vi "Set IPS Action.vi"(8 "error in (no error)":errorcluster, 10 "PSU Act Stat":T1="HOLD" caption="PSU Action Status", 11 "Instrument.Oxford1820 in":refnum<class "Instrument.Oxford1820.lvclass">) -> (0 "error out":errorcluster, 2 "Response":string, 3 "Instrument.Oxford1820 out":refnum<class "Instrument.Oxford1820.lvclass">)   [LabVIEW 2019, in "Instrument.Oxford1820.lvclass"]
uses:
  Instrument.Oxford1820.lvclass
  <instrlib>/Mercury iXX/Public/Libraries/Magnet/Controls/PSU Actions.ctl
  Instrument.Oxford1820.lvclass/Instrument.Oxford1820.ctl
  <instrlib>/Mercury iXX/Public/Libraries/Magnet/Open/Open Magnet Device.vi
  <instrlib>/Mercury iXX/Public/Libraries/Magnet/Configuration/Set/PSU Action Status (Set).vi
  <instrlib>/Mercury iXX/Public/Libraries/Magnet/Configuration/Read/PSU Action Status (Read).vi
  <instrlib>/Mercury iXX/Mercury iXX.lvlib
  <instrlib>/Mercury iXX/Public/Libraries/Magnet.lvlib
panel:
  out "Numeric":i32
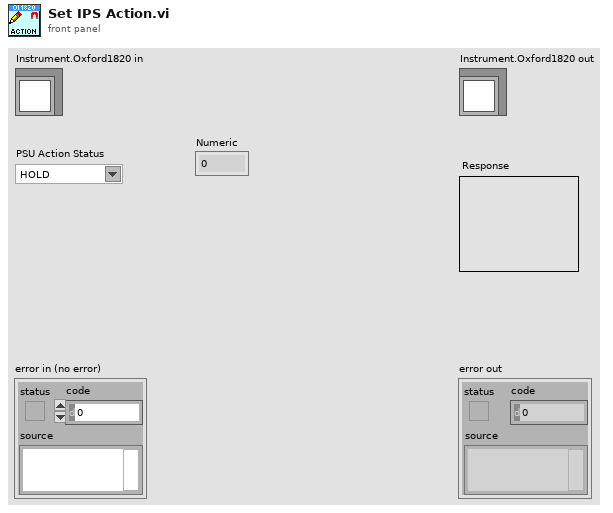
[diagram p1: front panel]
types:
  T1 = typedef "Mercury iXX.lvlib/Magnet.lvlib/PSU Actions.ctl" = string
  T2 = typedef "Mercury iXX.lvlib/Mercury Reference.ctl" = cluster{"Comms":refnum<visa-resource-name>, "Device ID":string[], "Comms Layer":T3, "Command":string, "Query reference":T4}
  T3 = typedef "Mercury iXX.lvlib/Comms Transport Layer.ctl" = enum16{"Ethernet TCP/IP", "USB", "ISOBus - RS-232", "GPIB"}
  T4 = typedef "Mercury iXX.lvlib/Query Dynamic Reference.ctl" = refnum<vi>
  T5 = typedef "Mercury iXX.lvlib/Response String.ctl" = string
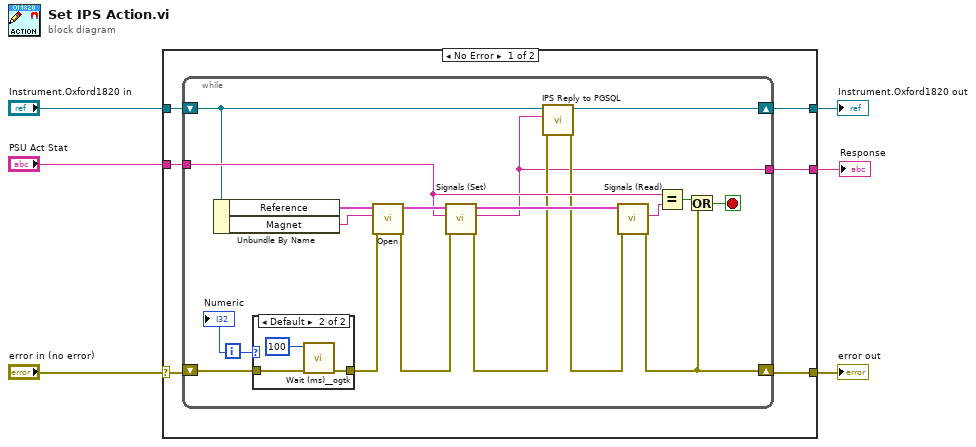
[diagram p0: block diagram]
diagram:
  n1 = case shown="No Error" "error in (no error)" {
    selector: "error in (no error)" -> [w11 w36]
    tunnel: [w9 w36] -> w5
    tunnel: [w7 w35] -> w3
    tunnel: "Instrument.Oxford1820 in" -> [w12 w35]
    tunnel: [w10 _] -> w2
    tunnel: "PSU Act Stat" -> [w8 _]
    frame No Error {
      n2 = while {
        tunnel: [w13] -> w10
        tunnel: w8 -> [w25]
        shift-right: [w20] -> w9
        shift-left: w11 -> [w23]
        shift-right: [w15] -> w7
        shift-left: w12 -> [w14]
        i -> [w22]
        stop <- w18 stop-if-true
        n3 = Unbundle By Name(w14) -> ("Reference"=w29:T2, "Magnet"=w30:string)
        n4 = case shown="Default" w22 {
          tunnel: w23 -> [w31 w34]
          tunnel: [w31 w33] -> w21
          frame 0 {
          }
          frame Default {
            n5 = call <userlib>:"Wait (ms)__ogtk.vi"("error in (no error)"=w34, "milliseconds to wait"=u32 100) -> ("error out"=w33:errorcluster)  [unwired: 8 in, 1 out]
          }
        }
        n6 = call-poly <instrlib>:"Open.vi"("error in (no error)"=w21, "Device Identifier"=w30, "Mercury Reference In"=w29) -> ("error out"=w27:errorcluster, "Mercury Reference Out"=w28:T2)  [unwired: 7 out]
        n7 = call-poly <instrlib>:"Signals (Set).vi"("error in"=w27, "PSU Act Stat"=w25, "Mercury Reference In"=w28) -> ("error out"=w17:errorcluster, "Response"=w13:T5, "Mercury Reference Out"=w26:T2)  [unwired: 1 in, 5 out]
        n8 = call "IPS Reply to PGSQL.vi"("error in (no error)"=w17, "Response"=w13, "Instrument.1820 in"=w14) -> ("error out"=w16:errorcluster, "Instrument.1820 out"=w15:refnum<class "Instrument.Oxford1820.lvclass">)  [unwired: 7 in]
        n9 = call-poly <instrlib>:"Signals (Read).vi"("error in"=w16, "Mercury Reference In"=w26) -> ("error out"=w20:errorcluster, "PSU Act Stat"=w24:T1)  [unwired: 1 in, 7 out]
        n10 = Equal?(x=w25, y=w24) -> (x = y?=w19:bool)
        n11 = Or(x=w19, y=w20) -> (x .or. y?=w18:bool)
        "Numeric" <- w22
      }
    }
    frame Error {
    }
  }
  "error out" <- w5
  "Instrument.Oxford1820 out" <- w3
  "Response" <- w2
